vi "Teleop.vi"(10 "Match Info":T1={"Autonomous Elapsed Seconds"=0.0, "TeleOp Elapsed Seconds"=0.0, "Disabled Elapsed Seconds"=0.0, "Visited Autonomous"=FALSE, "Visited TeleOp"=FALSE, "Visited Disabled"=FALSE, "Autonomous Settings"={"Autonomous Style"=enum."Independent", "VI Refnum"=refnum}}, 11 "Call Context":T2) -> ()   [LabVIEW 2015]
doc: "This VI is called for each TeleOp packet received from the DS where the robot is not disabled. It is often used to read from the joysticks and update I/O or to update setpoints for timed control loops. It should complete and return within 20 milliseconds or it may miss DS packets."
uses:
  <vilib>/Rock Robotics/WPI/DriverStation/WPI_DriverStationDerivedRobotMode.ctl
  <vilib>/Rock Robotics/WPI/DriverStation/WPI_DriverStationMatch Info.ctl
  <vilib>/Rock Robotics/WPI/Solenoid/WPI_SolenoidValue.ctl
  <vilib>/Rock Robotics/Network Tables/NT Read Boolean.vi
  <vilib>/Rock Robotics/Network Tables/NT Read Number.vi
  <vilib>/Rock Robotics/WPI/Utilities/WPI_GetSetVariantRefNum.vi
  <vilib>/addons/control/pid/pid.llb/PID (DBL).vi
  <vilib>/Rock Robotics/WPI/Solenoid/WPI_SolenoidGetEnum.vi
  <vilib>/Rock Robotics/WPI/Solenoid/WPI_SolenoidSetEnum.vi
  <vilib>/addons/control/pid/NI_PID_pid.lvlib
panel:
  out "Sample Slider 0":dbl(slide) scale=0.0..5.0
  out "Sample Boolean 1":bool
  out "Sample Boolean 0":bool
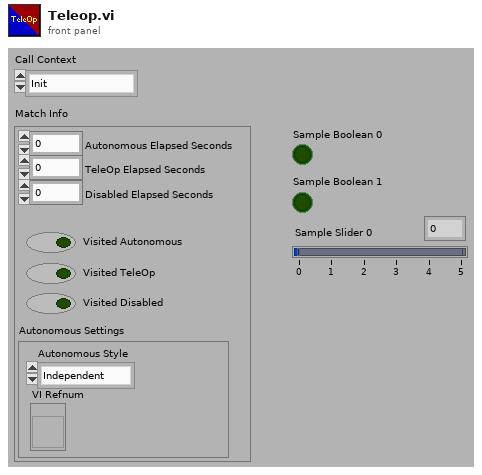
[diagram p1: front panel]
types:
  T1 = typedef "WPI_DriverStationMatch Info.ctl" = cluster{"Autonomous Elapsed Seconds":dbl, "TeleOp Elapsed Seconds":dbl, "Disabled Elapsed Seconds":dbl, "Visited Autonomous":bool, "Visited TeleOp":bool, "Visited Disabled":bool, "Autonomous Settings":cluster{"Autonomous Style":enum16{"Iterative", "Independent"}, "VI Refnum":refnum<vi>}}
  T2 = typedef "WPI_DriverStationDerivedRobotMode.ctl" = enum16{"Init", "Execute", "Stop"}
  T3 = typedef "WPI_SolenoidValue.ctl" = enum16{"Off", "On", "Forward", "Reverse"}
  T4 = typedef "WPI_JoystickDevRef.ctl" = cluster{"Device":T5}
  T5 = typedef "WPI_JoystickDeviceEnum.ctl" = enum16{"USB 0", "USB 1", "USB 2", "USB 3", "USB 4", "USB 5"}
  T6 = cluster{"Buttons[0]":bool, "Buttons[1]":bool, "Buttons[2]":bool, "Buttons[3]":bool, "Buttons[4]":bool, "Buttons[5]":bool, "Buttons[6]":bool, "Buttons[7]":bool, "Buttons[8]":bool}
  T7 = typedef "WPI_SolenoidDevRef.ctl" = cluster{"DevStatus":errorcluster, "Pneumatics Control Module":u8, "Forward Solenoid Channel":T8, "Reverse Solenoid Channel":T8}
  T8 = typedef "WPI_SolenoidChannel.ctl" = enum8{"Solenoid 0", "Solenoid 1", "Solenoid 2", "Solenoid 3", "Solenoid 4", "Solenoid 5", "Solenoid 6", "Solenoid 7", "Invalid"}
  T9 = cluster{"proportional gain (Kc)":dbl, "integral time (Ti, min)":dbl, "derivative time (Td, min)":dbl}
  T10 = cluster{"Axes[0]":dbl, "Axes[1]":dbl, "Axes[2]":dbl, "Axes[3]":dbl, "Axes[4]":dbl, "Axes[5]":dbl, "Axes[6]":dbl, "Axes[7]":dbl, "Axes[8]":dbl}
  T11 = typedef "WPI_RobotDriveDevRef.ctl" = cluster{"DevStatus":errorcluster, "Motors[]":T12[], "Square Inputs":bool, "Max Output":dbl}
  T12 = typedef "WPI_MotorControlDeviceRef.ctl" = cluster{"DeviceStatus":errorcluster, "Type":T13, "PWM":cluster{"PWM Channel":T14, "DeadBand":T15}, "CAN":cluster{"Device Number":u8, "Control Mode":T16, "Semaphore":T17, "Max Vout":dbl, "TalonSRX Control Mode":T18}, "Invert":bool}
  T13 = typedef "WPI_MotorControlType.ctl" = enum16{"PWM", "CAN", "CANTalonSRX"}
  T14 = typedef "FPGA_DIOPWMChannel.ctl" = enum8{"PWM 0", "PWM 1", "PWM 2", "PWM 3", "PWM 4", "PWM 5", "PWM 6", "PWM 7", "PWM 8", "PWM 9", "PWM MXP 0", "PWM MXP 1", "PWM MXP 2", "PWM MXP 3", "PWM MXP 4", "PWM MXP 5", "PWM MXP 6", "PWM MXP 7", "PWM MXP 8", "PWM MXP 9", "Invalid"}
  T15 = typedef "WPI_PWMDeadband.ctl" = cluster{"Name":string, "maxPositivePwm":i32, "minPositivePwm":i32, "centerPwm":i32, "maxNegativePwm":i32, "minNegativePwm":i32, "angularRange":u16}
  T16 = typedef "WPI_CANJaguar_ControlMode.ctl" = enum8{"Percent VBus", "Current", "Speed", "Position", "Voltage"}
  T17 = typedef "Semaphore RefNum" = refnum<k1>
  T18 = typedef "WPI_CANTalonSRX_APIControlMode.ctl" = enum8{"Percent VBus", "Speed", "Position", "Slave", "Unchanged / Invalid", "Voltage Compensation", "Current", "Motion Profile"}
  T19 = typedef "WPI_EncoderDevRef.ctl" = cluster{"DevStatus":errorcluster, "EncoderIndex":T20, "CounterIndex":T21, "DistancePerCount":dbl, "Decoding Type":T22}
  T20 = typedef "FPGA_EncoderIdx.ctl" = enum8{"Enc 0", "Enc 1", "Enc 2", "Enc 3", "Enc 4", "Enc 5", "Enc 6", "Enc 7", "Invalid"}
  T21 = typedef "FPGA_CounterCtrSystemIndex.ctl" = enum8{"Ctr 0", "Ctr 1", "Ctr 2", "Ctr 3", "Ctr 4", "Ctr 5", "Ctr 6", "Ctr 7", "Invalid"}
  T22 = typedef "WPI_EncoderType.ctl" = enum16{"1x", "2x", "4x"}
  T23 = typedef "WPI_CompressorDevRef.ctl" = cluster{"DevStatus":errorcluster, "Pneumatics Control Module":u8}
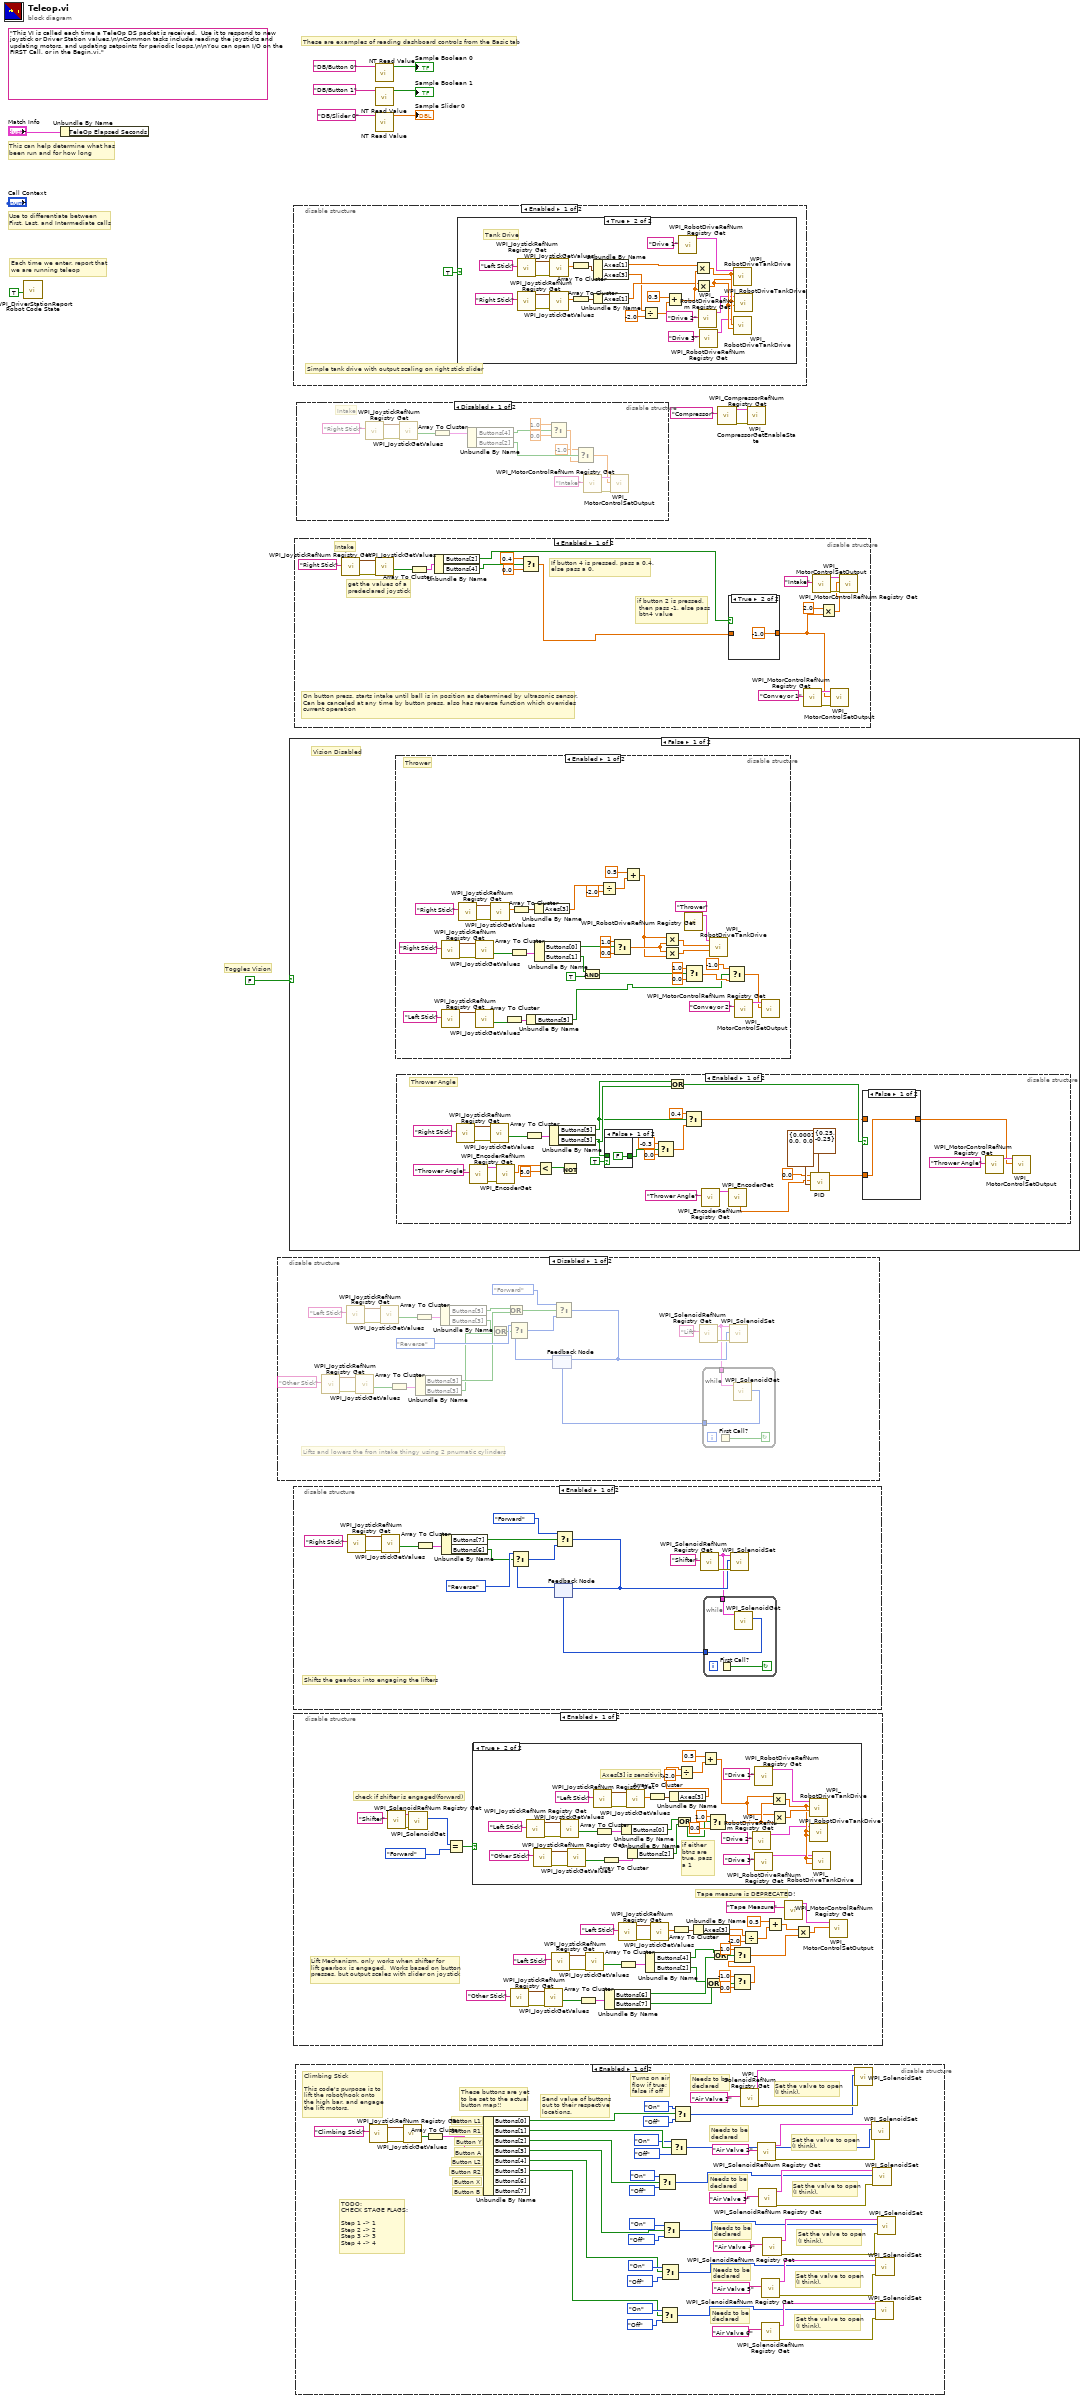
[diagram p0: block diagram]
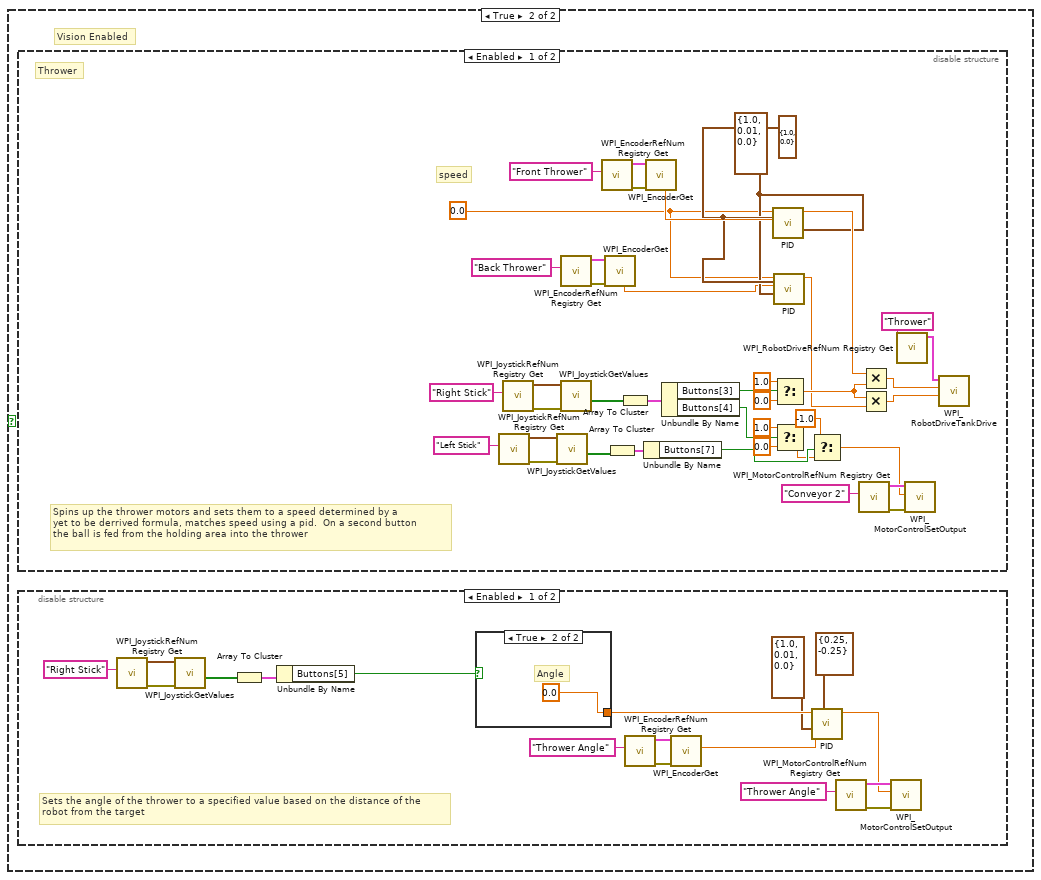
[diagram p11: hidden frame]
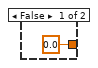
[diagram p12: hidden frame]
diagram:
  (unwired) "This VI is called each time a TeleOp DS packet is received.  Use it to respond to new joystick or Driver Station values.\n\nCommon tasks include reading the joysticks and updating motors, and updating setpoints for periodic loops.\n\nYou can open I/O on the FIRST Call, or in the Begin.vi."
  # "Toggles Vision"
  # "These are examples of reading dashboard controls from the Basic tab"
  # "Each time we enter, report that\nwe are running teleop"
  # "Use to differentiate between\nFirst, Last, and Intermediate calls"
  # "This can help determine what has\nbeen run and for how long"
  n1 = call <vilib>:"WPI_DriverStationReport Robot Code State.vi"("TeleOp"=TRUE ("Autonomous")) -> ()  [unwired: 10 in, 1 out]
  n2 = Unbundle By Name("Match Info") -> ()  [unwired: 1 out]
  n3 = disable-structure shown="Disabled" {
    frame Disabled {
      # "Lifts and lowers the fron intake thingy using 2 pnumatic cylinders"
      n4 = call <vilib>:"WPI_JoystickRefNum Registry Get.vi"("refnum name"="Other Stick") -> ("error out"=w23:errorcluster, "JoystickDevRef"=w22:T4)  [unwired: 9 in]
      n5 = call <vilib>:"WPI_JoystickRefNum Registry Get.vi"("refnum name"="Left Stick") -> ("error out"=w37:errorcluster, "JoystickDevRef"=w36:T4)  [unwired: 9 in]
      n6 = call <vilib>:"WPI_JoystickGetValues.vi"("error in (no error)"=w23, "JoystickDevRef"=w22) -> ("Buttons"=w20:bool[])  [unwired: 5 in, 4 out]
      n7 = call <vilib>:"WPI_JoystickGetValues.vi"("error in (no error)"=w37, "JoystickDevRef"=w36) -> ("Buttons"=w34:bool[])  [unwired: 5 in, 4 out]
      n8 = Array To Cluster(array=w20) -> (cluster=w19:T6)
      n9 = Array To Cluster(array=w34) -> (cluster=w33:T6)
      n10 = Unbundle By Name(w19) -> ("Buttons[5]"=w16:bool, "Buttons[3]"=w14:bool)
      n11 = Unbundle By Name(w33) -> ("Buttons[5]"=w18:bool, "Buttons[3]"=w13:bool)
      n12 = Or(x=w13, y=w14) -> (x .or. y?=w15:bool)
      n13 = Or(x=w18, y=w16) -> (x .or. y?=w17:bool)
      n14 = call <vilib>:"WPI_SolenoidRefNum Registry Get.vi"("refnum name"="Lift") -> ("error out"=w31:errorcluster, "SolenoidDevRef"=w25:T7)  [unwired: 9 in]
      n15 = while {
        tunnel: w25 -> [w39]
        tunnel: [w38] -> w24
        stop <- w40 continue-if-true
        n16 = First Call?() -> (First Call?: T/F=w40:bool)
        n17 = call-poly <vilib>:"WPI_SolenoidGet.vi"("SolenoidDevRef"=w39) -> ("Value"=w38:T3)  [unwired: 8 in, 2 out]
      }
      n18 = feedback #1(w24) -> (w26:T3)
      n19 = Select(t=WPI_SolenoidValue."Reverse" ("Value"), s=w15, f=w26) -> (s? t:f=w28:T3)
      n20 = Select(t=WPI_SolenoidValue."Forward" ("Value"), s=w17, f=w28) -> (s? t:f=w27:T3)
      n21 = feedback-in #1(w27) -> ()
      n22 = call-poly <vilib>:"WPI_SolenoidSet.vi"("error in (no error)"=w31, "Value"=w27, "SolenoidDevRef"=w25) -> ()  [unwired: 7 in, 2 out]
    }
    frame Enabled {
    }
  }
  n23 = case shown="False" FALSE {
    frame False {
      # "Vision Disabled"
      n24 = disable-structure shown="Enabled" {
        frame Enabled {
          # "Thrower"
          n25 = call <vilib>:"WPI_JoystickRefNum Registry Get.vi"("refnum name"="Right Stick") -> ("error out"=w113:errorcluster, "JoystickDevRef"=w112:T4)  [unwired: 9 in]
          n26 = call <vilib>:"WPI_JoystickRefNum Registry Get.vi"("refnum name"="Left Stick") -> ("JoystickDevRef"=w84:T4)  [unwired: 9 in, 1 out]
          n27 = call <vilib>:"WPI_JoystickRefNum Registry Get.vi"("refnum name"="Right Stick") -> ("error out"=w96:errorcluster, "JoystickDevRef"=w95:T4)  [unwired: 9 in]
          n28 = call <vilib>:"WPI_JoystickGetValues.vi"("error in (no error)"=w113, "JoystickDevRef"=w112) -> ("Buttons"=w110:bool[])  [unwired: 5 in, 4 out]
          n29 = call <vilib>:"WPI_JoystickGetValues.vi"("JoystickDevRef"=w84) -> ("Buttons"=w82:bool[])  [unwired: 6 in, 4 out]
          n30 = call <vilib>:"WPI_JoystickGetValues.vi"("error in (no error)"=w96, "JoystickDevRef"=w95) -> ("Axes"=w94:dbl[])  [unwired: 5 in, 4 out]
          n31 = Array To Cluster(array=w82) -> (cluster=w81:T6)
          n32 = Array To Cluster(array=w110) -> (cluster=w109:T6)
          n33 = Array To Cluster(array=w94) -> (cluster=w93:T10)
          n34 = Unbundle By Name(w81) -> ("Buttons[5]"=w76:bool)
          n35 = Unbundle By Name(w93) -> ("Axes[3]"=w89:dbl)
          n36 = Unbundle By Name(w109) -> ("Buttons[0]"=w108:bool, "Buttons[1]"=w86:bool)
          n37 = And(x=w86, y=TRUE) -> (x .and. y?=w80:bool)
          n38 = Divide(x=w89, y=-2.0) -> (x/y=w91:dbl)
          n39 = Select(t=1.0, s=w108, f=0.0) -> (s? t:f=w105:dbl)
          n40 = Add(x=0.5, y=w91) -> (x+y=w87:dbl)
          n41 = Multiply(x=w87, y=w105) -> (x*y=w103:dbl)
          n42 = Multiply(x=w105, y=w87) -> (x*y=w104:dbl)
          n43 = call <vilib>:"WPI_RobotDriveRefNum Registry Get.vi"("refnum name"="Thrower") -> ("RobotDriveDevRef"=w102:T11)  [unwired: 9 in, 1 out]
          n44 = Select(t=1.0, s=w80, f=0.0) -> (s? t:f=w79:dbl)
          n45 = call <vilib>:"WPI_RobotDriveTankDrive.vi"("Right axis value"=w104, "Left axis value"=w103, "RobotDriveDevRef"=w102) -> ()  [unwired: 6 in, 3 out]
          n46 = Select(t=-1.0, s=w76, f=w79) -> (s? t:f=w77:dbl)
          n47 = call <vilib>:"WPI_MotorControlRefNum Registry Get.vi"("refnum name"="Conveyor 2") -> ("MotorControlDevRef"=w100:T12)  [unwired: 9 in, 1 out]
          n48 = call <vilib>:"WPI_MotorControlSetOutput.vi"("Output"=w77, "MotorControlDevRef"=w100) -> ()  [unwired: 7 in, 3 out]
        }
        frame Disabled {
        }
      }
      n49 = disable-structure shown="Enabled" {
        frame Enabled {
          # "Thrower Angle"
          n50 = call <vilib>:"WPI_JoystickRefNum Registry Get.vi"("refnum name"="Right Stick") -> ("error out"=w71:errorcluster, "JoystickDevRef"=w70:T4)  [unwired: 9 in]
          n51 = call <vilib>:"WPI_EncoderRefNum Registry Get.vi"("refnum name"="Thrower Angle") -> ("error out"=w63:errorcluster, "EncoderDevRef"=w61:T19)  [unwired: 9 in]
          n52 = call <vilib>:"WPI_JoystickGetValues.vi"("error in (no error)"=w71, "JoystickDevRef"=w70) -> ("Buttons"=w68:bool[])  [unwired: 5 in, 4 out]
          n53 = call <vilib>:"WPI_EncoderGet.vi"("error in (no error)"=w63, "EncoderDevRef"=w61) -> ("Distance"=w60:dbl)  [unwired: 4 in, 5 out]
          n54 = Array To Cluster(array=w68) -> (cluster=w67:T6)
          n55 = Less?(x=w60, y=5.0) -> (x < y?=w58:bool)
          n56 = Unbundle By Name(w67) -> ("Buttons[5]"=w47:bool, "Buttons[3]"=w48:bool)
          n57 = Not(x=w58) -> ()  [unwired: 1 out]
          n58 = case shown="False" TRUE {
            tunnel: w48 -> [_ w75]
            tunnel: [FALSE ("Buttons[6]") w75] -> w57
            frame False {
            }
            frame True {
            }
          }
          n59 = Select(t=-0.3, s=w57, f=0.0) -> (s? t:f=w56:dbl)
          n60 = Or(x=w47, y=w48) -> (x .or. y?=w46:bool)
          n61 = Select(t=0.4, s=w47, f=w56) -> (s? t:f=w45:dbl)
          n62 = call <vilib>:"WPI_EncoderRefNum Registry Get.vi"("refnum name"="Thrower Angle") -> ("EncoderDevRef"=w52:T19)  [unwired: 9 in, 1 out]
          n63 = call <vilib>:"WPI_EncoderGet.vi"("EncoderDevRef"=w52) -> ("Rate"=w41:dbl)  [unwired: 5 in, 5 out]
          n64 = call-poly <vilib>:"PID.vi"("output range"=cluster{"output high":dbl, "output low":dbl} {"output high"=0.25, "output low"=-0.25}, "PID gains"=T9 {"proportional gain (Kc)"=0.0001, "integral time (Ti, min)"=0.0, "derivative time (Td, min)"=0.0}, "process variable"=w41, "setpoint"=0.0) -> ("output"=w43:dbl)  [unwired: 6 in, 1 out]
          n65 = case shown="False" w46 {
            tunnel: [w72 w73] -> w44
            tunnel: w45 -> [_ w73]
            tunnel: w43 -> [w72 _]
            frame False {
            }
            frame True {
            }
          }
          n66 = call <vilib>:"WPI_MotorControlRefNum Registry Get.vi"("refnum name"="Thrower Angle") -> ("MotorControlDevRef"=w54:T12)  [unwired: 9 in, 1 out]
          n67 = call <vilib>:"WPI_MotorControlSetOutput.vi"("Output"=w44, "MotorControlDevRef"=w54) -> ()  [unwired: 7 in, 3 out]
        }
        frame Disabled {
        }
      }
    }
    frame True {
      # "Vision Enabled"
      n68 = disable-structure shown="Enabled" {
        frame Enabled {
          w153 = 0.0 ("setpoint")
          w154 = T9 {"proportional gain (Kc)"=1.0, "integral time (Ti, min)"=0.01, "derivative time (Td, min)"=0.0} ("PID gains")
          w155 = cluster{"output high":dbl, "output low":dbl} {"output high"=1.0, "output low"=0.0} ("output range")
          # "Spins up the thrower motors and sets them to a speed determined by a \nyet to be derrived formula, matches speed using a pid.  On a second button\nthe ball is fed from the holding area into the thrower"
          # "Thrower"
          # "speed"
          n69 = call <vilib>:"WPI_JoystickRefNum Registry Get.vi"("refnum name"="Left Stick") -> ("error out"=w141:errorcluster, "JoystickDevRef"=w140:T4)  [unwired: 9 in]
          n70 = call <vilib>:"WPI_JoystickRefNum Registry Get.vi"("refnum name"="Right Stick") -> ("error out"=w173:errorcluster, "JoystickDevRef"=w172:T4)  [unwired: 9 in]
          n71 = call <vilib>:"WPI_JoystickGetValues.vi"("error in (no error)"=w141, "JoystickDevRef"=w140) -> ("Buttons"=w138:bool[])  [unwired: 5 in, 4 out]
          n72 = call <vilib>:"WPI_EncoderRefNum Registry Get.vi"("refnum name"="Back Thrower") -> ("error out"=w152:errorcluster, "EncoderDevRef"=w151:T19)  [unwired: 9 in]
          n73 = call <vilib>:"WPI_JoystickGetValues.vi"("error in (no error)"=w173, "JoystickDevRef"=w172) -> ("Buttons"=w170:bool[])  [unwired: 5 in, 4 out]
          n74 = call <vilib>:"WPI_EncoderRefNum Registry Get.vi"("refnum name"="Front Thrower") -> ("error out"=w160:errorcluster, "EncoderDevRef"=w159:T19)  [unwired: 9 in]
          n75 = call <vilib>:"WPI_EncoderGet.vi"("error in (no error)"=w152, "EncoderDevRef"=w151) -> ("Rate"=w149:dbl)  [unwired: 4 in, 5 out]
          n76 = Array To Cluster(array=w138) -> (cluster=w137:T6)
          n77 = Array To Cluster(array=w170) -> (cluster=w169:T6)
          n78 = Unbundle By Name(w137) -> ("Buttons[7]"=w136:bool)
          n79 = call <vilib>:"WPI_EncoderGet.vi"("error in (no error)"=w160, "EncoderDevRef"=w159) -> ("Rate"=w157:dbl)  [unwired: 4 in, 5 out]
          n80 = Unbundle By Name(w169) -> ("Buttons[3]"=w168:bool, "Buttons[4]"=w143:bool)
          n81 = call-poly <vilib>:"PID.vi"("output range"=w155, "PID gains"=w154, "process variable"=w157, "setpoint"=w153) -> ("output"=w156:dbl)  [unwired: 6 in, 1 out]
          n82 = call-poly <vilib>:"PID.vi"("output range"=w155, "PID gains"=w154, "process variable"=w149, "setpoint"=w153) -> ("output"=w148:dbl)  [unwired: 6 in, 1 out]
          n83 = Select(t=1.0, s=w168, f=0.0) -> (s? t:f=w165:dbl)
          n84 = Select(t=1.0, s=w143, f=0.0) -> (s? t:f=w135:dbl)
          n85 = Select(t=-1.0, s=w136, f=w135) -> (s? t:f=w133:dbl)
          n86 = call <vilib>:"WPI_MotorControlRefNum Registry Get.vi"("refnum name"="Conveyor 2") -> ("error out"=w147:errorcluster, "MotorControlDevRef"=w145:T12)  [unwired: 9 in]
          n87 = Multiply(x=w156, y=w165) -> (x*y=w163:dbl)
          n88 = Multiply(x=w165, y=w148) -> (x*y=w164:dbl)
          n89 = call <vilib>:"WPI_RobotDriveRefNum Registry Get.vi"("refnum name"="Thrower") -> ("RobotDriveDevRef"=w162:T11)  [unwired: 9 in, 1 out]
          n90 = call <vilib>:"WPI_MotorControlSetOutput.vi"("error in (no error)"=w147, "Output"=w133, "MotorControlDevRef"=w145) -> ()  [unwired: 6 in, 3 out]
          n91 = call <vilib>:"WPI_RobotDriveTankDrive.vi"("Right axis value"=w164, "Left axis value"=w163, "RobotDriveDevRef"=w162) -> ()  [unwired: 6 in, 3 out]
        }
        frame Disabled {
        }
      }
      n92 = disable-structure shown="Enabled" {
        frame Enabled {
          # "Sets the angle of the thrower to a specified value based on the distance of the\nrobot from the target"
          n93 = call <vilib>:"WPI_JoystickRefNum Registry Get.vi"("refnum name"="Right Stick") -> ("error out"=w120:errorcluster, "JoystickDevRef"=w119:T4)  [unwired: 9 in]
          n94 = call <vilib>:"WPI_JoystickGetValues.vi"("error in (no error)"=w120, "JoystickDevRef"=w119) -> ("Buttons"=w117:bool[])  [unwired: 5 in, 4 out]
          n95 = Array To Cluster(array=w117) -> (cluster=w116:T6)
          n96 = Unbundle By Name(w116) -> ("Buttons[5]"=w115:bool)
          n97 = case shown="True" w115 {
            tunnel: [0.0 ("setpoint") 0.0 ("setpoint")] -> w128
            frame False {
            }
            frame True {
              # "Angle"
            }
          }
          n98 = call <vilib>:"WPI_EncoderRefNum Registry Get.vi"("refnum name"="Thrower Angle") -> ("error out"=w130:errorcluster, "EncoderDevRef"=w129:T19)  [unwired: 9 in]
          n99 = call <vilib>:"WPI_EncoderGet.vi"("error in (no error)"=w130, "EncoderDevRef"=w129) -> ("Distance"=w127:dbl)  [unwired: 4 in, 5 out]
          n100 = call-poly <vilib>:"PID.vi"("output range"=cluster{"output high":dbl, "output low":dbl} {"output high"=0.25, "output low"=-0.25}, "PID gains"=T9 {"proportional gain (Kc)"=1.0, "integral time (Ti, min)"=0.01, "derivative time (Td, min)"=0.0}, "process variable"=w127, "setpoint"=w128) -> ("output"=w121:dbl)  [unwired: 6 in, 1 out]
          n101 = call <vilib>:"WPI_MotorControlRefNum Registry Get.vi"("refnum name"="Thrower Angle") -> ("error out"=w123:errorcluster, "MotorControlDevRef"=w122:T12)  [unwired: 9 in]
          n102 = call <vilib>:"WPI_MotorControlSetOutput.vi"("error in (no error)"=w123, "Output"=w121, "MotorControlDevRef"=w122) -> ()  [unwired: 6 in, 3 out]
        }
        frame Disabled {
        }
      }
    }
  }
  n103 = disable-structure shown="Enabled" {
    frame Enabled {
      # "Shifts the gearbox into engaging the lifters"
      n104 = call <vilib>:"WPI_JoystickRefNum Registry Get.vi"("refnum name"="Right Stick") -> ("error out"=w189:errorcluster, "JoystickDevRef"=w188:T4)  [unwired: 9 in]
      n105 = call <vilib>:"WPI_JoystickGetValues.vi"("error in (no error)"=w189, "JoystickDevRef"=w188) -> ("Buttons"=w186:bool[])  [unwired: 5 in, 4 out]
      n106 = Array To Cluster(array=w186) -> (cluster=w185:T6)
      n107 = Unbundle By Name(w185) -> ("Buttons[7]"=w179:bool, "Buttons[6]"=w180:bool)
      n108 = call <vilib>:"WPI_SolenoidRefNum Registry Get.vi"("refnum name"="Shifter") -> ("error out"=w183:errorcluster, "SolenoidDevRef"=w175:T7)  [unwired: 9 in]
      n109 = while {
        tunnel: w175 -> [w191]
        tunnel: [w190] -> w174
        stop <- w192 continue-if-true
        n110 = First Call?() -> (First Call?: T/F=w192:bool)
        n111 = call-poly <vilib>:"WPI_SolenoidGet.vi"("SolenoidDevRef"=w191) -> ("Value"=w190:T3)  [unwired: 8 in, 2 out]
      }
      n112 = feedback #2(w174) -> (w176:T3)
      n113 = Select(t=WPI_SolenoidValue."Reverse" ("Value"), s=w180, f=w176) -> (s? t:f=w178:T3)
      n114 = Select(t=WPI_SolenoidValue."Forward" ("Value"), s=w179, f=w178) -> (s? t:f=w177:T3)
      n115 = feedback-in #2(w177) -> ()
      n116 = call-poly <vilib>:"WPI_SolenoidSet.vi"("error in (no error)"=w183, "Value"=w177, "SolenoidDevRef"=w175) -> ()  [unwired: 7 in, 2 out]
    }
    frame Disabled {
    }
  }
  n117 = disable-structure shown="Enabled" {
    frame Enabled {
      # "Simple tank drive with output scaling on right stick slider"
      n118 = case shown="True" TRUE {
        frame False {
        }
        frame True {
          # "Tank Drive"
          n119 = call <vilib>:"WPI_JoystickRefNum Registry Get.vi"("refnum name"="Left Stick") -> ("error out"=w217:errorcluster, "JoystickDevRef"=w216:T4)  [unwired: 9 in]
          n120 = call <vilib>:"WPI_JoystickRefNum Registry Get.vi"("refnum name"="Right Stick") -> ("error out"=w212:errorcluster, "JoystickDevRef"=w211:T4)  [unwired: 9 in]
          n121 = call <vilib>:"WPI_JoystickGetValues.vi"("error in (no error)"=w217, "JoystickDevRef"=w216) -> ("Axes"=w215:dbl[])  [unwired: 5 in, 4 out]
          n122 = call <vilib>:"WPI_JoystickGetValues.vi"("error in (no error)"=w212, "JoystickDevRef"=w211) -> ("Axes"=w210:dbl[])  [unwired: 5 in, 4 out]
          n123 = Array To Cluster(array=w215) -> (cluster=w214:T10)
          n124 = Array To Cluster(array=w210) -> (cluster=w209:T10)
          n125 = Unbundle By Name(w214) -> ("Axes[1]"=w203:dbl, "Axes[3]"=w194:dbl)
          n126 = Unbundle By Name(w209) -> ("Axes[1]"=w204:dbl)
          n127 = Divide(x=w194, y=-2.0) -> (x/y=w207:dbl)
          n128 = Add(x=0.5, y=w207) -> (x+y=w205:dbl)
          n129 = call <vilib>:"WPI_RobotDriveRefNum Registry Get.vi"("refnum name"="Drive 1") -> ("RobotDriveDevRef"=w202:T11)  [unwired: 9 in, 1 out]
          n130 = Multiply(x=w203, y=w205) -> (x*y=w200:dbl)
          n131 = Multiply(x=w204, y=w205) -> (x*y=w199:dbl)
          n132 = call <vilib>:"WPI_RobotDriveRefNum Registry Get.vi"("refnum name"="Drive 2") -> ("RobotDriveDevRef"=w197:T11)  [unwired: 9 in, 1 out]
          n133 = call <vilib>:"WPI_RobotDriveRefNum Registry Get.vi"("refnum name"="Drive 3") -> ("RobotDriveDevRef"=w195:T11)  [unwired: 9 in, 1 out]
          n134 = call <vilib>:"WPI_RobotDriveTankDrive.vi"("Right axis value"=w199, "Left axis value"=w200, "RobotDriveDevRef"=w202) -> ()  [unwired: 6 in, 3 out]
          n135 = call <vilib>:"WPI_RobotDriveTankDrive.vi"("Right axis value"=w199, "Left axis value"=w200, "RobotDriveDevRef"=w195) -> ()  [unwired: 6 in, 3 out]
          n136 = call <vilib>:"WPI_RobotDriveTankDrive.vi"("Right axis value"=w199, "Left axis value"=w200, "RobotDriveDevRef"=w197) -> ()  [unwired: 6 in, 3 out]
        }
      }
    }
    frame Disabled {
    }
  }
  n137 = disable-structure shown="Enabled" {
    frame Enabled {
      # "Tape measure is DEPRECATED!"
      # "check if shifter is engaged(forward)"
      # "Lift Mechanism, only works when shifter for\nlift gearbox is engaged.  Works based on button\npresses, but output scales with slider on joystick"
      n138 = call <vilib>:"WPI_SolenoidRefNum Registry Get.vi"("refnum name"="Shifter") -> ("error out"=w257:errorcluster, "SolenoidDevRef"=w256:T7)  [unwired: 9 in]
      n139 = call-poly <vilib>:"WPI_SolenoidGet.vi"("error in (no error)"=w257, "SolenoidDevRef"=w256) -> ("Value"=w254:T3)  [unwired: 7 in, 2 out]
      n140 = Equal?(x=w254, y=WPI_SolenoidValue."Forward") -> (x = y?=w255:bool)
      n141 = case shown="True" w255 {
        frame False {
        }
        frame True {
          # "Axes[3] is sensitivity"
          # "if either btns are true, pass a 1"
          n142 = call <vilib>:"WPI_JoystickRefNum Registry Get.vi"("refnum name"="Left Stick") -> ("error out"=w288:errorcluster, "JoystickDevRef"=w289:T4)  [unwired: 9 in]
          n143 = call <vilib>:"WPI_JoystickRefNum Registry Get.vi"("refnum name"="Other Stick") -> ("error out"=w271:errorcluster, "JoystickDevRef"=w270:T4)  [unwired: 9 in]
          n144 = call <vilib>:"WPI_JoystickGetValues.vi"("error in (no error)"=w288, "JoystickDevRef"=w289) -> ("Buttons"=w291:bool[])  [unwired: 5 in, 4 out]
          n145 = call <vilib>:"WPI_JoystickGetValues.vi"("error in (no error)"=w271, "JoystickDevRef"=w270) -> ("Buttons"=w268:bool[])  [unwired: 5 in, 4 out]
          n146 = call <vilib>:"WPI_JoystickRefNum Registry Get.vi"("refnum name"="Left Stick") -> ("error out"=w286:errorcluster, "JoystickDevRef"=w285:T4)  [unwired: 9 in]
          n147 = Array To Cluster(array=w291) -> (cluster=w292:T6)
          n148 = Array To Cluster(array=w268) -> (cluster=w267:T6)
          n149 = Unbundle By Name(w292) -> ("Buttons[0]"=w265:bool)
          n150 = call <vilib>:"WPI_JoystickGetValues.vi"("error in (no error)"=w286, "JoystickDevRef"=w285) -> ("Axes"=w284:dbl[])  [unwired: 5 in, 4 out]
          n151 = Unbundle By Name(w267) -> ("Buttons[2]"=w264:bool)
          n152 = Array To Cluster(array=w284) -> (cluster=w283:T10)
          n153 = Unbundle By Name(w283) -> ("Axes[3]"=w274:dbl)
          n154 = Or(x=w265, y=w264) -> (x .or. y?=w266:bool)
          n155 = Divide(x=w274, y=-2.0) -> (x/y=w277:dbl)
          n156 = Add(x=0.5, y=w277) -> (x+y=w273:dbl)
          n157 = Select(t=1.0, s=w266, f=0.0) -> (s? t:f=w278:dbl)
          n158 = call <vilib>:"WPI_RobotDriveRefNum Registry Get.vi"("refnum name"="Drive 2") -> ("RobotDriveDevRef"=w259:T11)  [unwired: 9 in, 1 out]
          n159 = call <vilib>:"WPI_RobotDriveRefNum Registry Get.vi"("refnum name"="Drive 1") -> ("RobotDriveDevRef"=w282:T11)  [unwired: 9 in, 1 out]
          n160 = call <vilib>:"WPI_RobotDriveRefNum Registry Get.vi"("refnum name"="Drive 3") -> ("RobotDriveDevRef"=w260:T11)  [unwired: 9 in, 1 out]
          n161 = Multiply(x=w273, y=w278) -> (x*y=w261:dbl)
          n162 = Multiply(x=w273, y=w278) -> (x*y=w280:dbl)
          n163 = call <vilib>:"WPI_RobotDriveTankDrive.vi"("Right axis value"=w280, "Left axis value"=w261, "RobotDriveDevRef"=w282) -> ()  [unwired: 6 in, 3 out]
          n164 = call <vilib>:"WPI_RobotDriveTankDrive.vi"("Right axis value"=w261, "Left axis value"=w261, "RobotDriveDevRef"=w259) -> ()  [unwired: 6 in, 3 out]
          n165 = call <vilib>:"WPI_RobotDriveTankDrive.vi"("Right axis value"=w261, "Left axis value"=w261, "RobotDriveDevRef"=w260) -> ()  [unwired: 6 in, 3 out]
        }
      }
      n166 = call <vilib>:"WPI_JoystickRefNum Registry Get.vi"("refnum name"="Other Stick") -> ("error out"=w229:errorcluster, "JoystickDevRef"=w220:T4)  [unwired: 9 in]
      n167 = call <vilib>:"WPI_JoystickGetValues.vi"("error in (no error)"=w229, "JoystickDevRef"=w220) -> ("Buttons"=w227:bool[])  [unwired: 5 in, 4 out]
      n168 = call <vilib>:"WPI_JoystickRefNum Registry Get.vi"("refnum name"="Left Stick") -> ("error out"=w248:errorcluster, "JoystickDevRef"=w249:T4)  [unwired: 9 in]
      n169 = Array To Cluster(array=w227) -> (cluster=w226:T6)
      n170 = call <vilib>:"WPI_JoystickGetValues.vi"("error in (no error)"=w248, "JoystickDevRef"=w249) -> ("Buttons"=w251:bool[])  [unwired: 5 in, 4 out]
      n171 = Unbundle By Name(w226) -> ("Buttons[6]"=w224:bool, "Buttons[7]"=w221:bool)
      n172 = call <vilib>:"WPI_JoystickRefNum Registry Get.vi"("refnum name"="Left Stick") -> ("error out"=w246:errorcluster, "JoystickDevRef"=w245:T4)  [unwired: 9 in]
      n173 = Array To Cluster(array=w251) -> (cluster=w252:T6)
      n174 = Unbundle By Name(w252) -> ("Buttons[4]"=w225:bool, "Buttons[2]"=w222:bool)
      n175 = call <vilib>:"WPI_JoystickGetValues.vi"("error in (no error)"=w246, "JoystickDevRef"=w245) -> ("Axes"=w244:dbl[])  [unwired: 5 in, 4 out]
      n176 = Array To Cluster(array=w244) -> (cluster=w243:T10)
      n177 = Unbundle By Name(w243) -> ("Axes[3]"=w232:dbl)
      n178 = Or(x=w222, y=w221) -> (x .or. y?=w223:bool)
      n179 = Or(x=w225, y=w224) -> (x .or. y?=w219:bool)
      n180 = Select(t=-1.0, s=w223, f=0.0) -> (s? t:f=w240:dbl)
      n181 = Select(t=1.0, s=w219, f=w240) -> (s? t:f=w239:dbl)
      n182 = Divide(x=w232, y=-2.0) -> (x/y=w235:dbl)
      n183 = Add(x=0.5, y=w235) -> (x+y=w231:dbl)
      n184 = call <vilib>:"WPI_MotorControlRefNum Registry Get.vi"("refnum name"="Tape Measure") -> ("MotorControlDevRef"=w237:T12)  [unwired: 9 in, 1 out]
      n185 = Multiply(x=w231, y=w239) -> (x*y=w236:dbl)
      n186 = call <vilib>:"WPI_MotorControlSetOutput.vi"("Output"=w236, "MotorControlDevRef"=w237) -> ()  [unwired: 7 in, 3 out]
    }
    frame Disabled {
    }
  }
  n187 = disable-structure shown="Enabled" {
    frame Enabled {
      # "if button 2 is pressed,\n then pass -1, else pass\n btn4 value"
      # "get the values of a\npredeclared joystick"
      # "If button 4 is pressed, pass a 0.4.\nelse pass a 0."
      # "On button press, starts intake until ball is in position as determined by ultrasonic sensor.\nCan be canceled at any time by button press, also has reverse function which overrides \ncurrent operation"
      # "Intake"
      n188 = call <vilib>:"WPI_JoystickRefNum Registry Get.vi"("refnum name"="Right Stick") -> ("error out"=w311:errorcluster, "JoystickDevRef"=w310:T4)  [unwired: 9 in]
      n189 = call <vilib>:"WPI_JoystickGetValues.vi"("error in (no error)"=w311, "JoystickDevRef"=w310) -> ("Buttons"=w308:bool[])  [unwired: 5 in, 4 out]
      n190 = Array To Cluster(array=w308) -> (cluster=w307:T6)
      n191 = Unbundle By Name(w307) -> ("Buttons[2]"=w302:bool, "Buttons[4]"=w306:bool)
      n192 = Select(t=0.4, s=w306, f=0.0) -> (s? t:f=w293:dbl)
      n193 = case shown="True" w302 {
        tunnel: [w312 -1.0 ("t")] -> w296
        tunnel: w293 -> [w312 _]
        frame False {
        }
        frame True {
        }
      }
      n194 = call <vilib>:"WPI_MotorControlRefNum Registry Get.vi"("refnum name"="Conveyor 1") -> ("error out"=w305:errorcluster, "MotorControlDevRef"=w303:T12)  [unwired: 9 in]
      n195 = call <vilib>:"WPI_MotorControlRefNum Registry Get.vi"("refnum name"="Intake") -> ("error out"=w298:errorcluster, "MotorControlDevRef"=w297:T12)  [unwired: 9 in]
      n196 = Multiply(x=2.0, y=w296) -> (x*y=w294:dbl)
      n197 = call <vilib>:"WPI_MotorControlSetOutput.vi"("error in (no error)"=w305, "Output"=w296, "MotorControlDevRef"=w303) -> ()  [unwired: 6 in, 3 out]
      n198 = call <vilib>:"WPI_MotorControlSetOutput.vi"("error in (no error)"=w298, "Output"=w294, "MotorControlDevRef"=w297) -> ()  [unwired: 6 in, 3 out]
    }
    frame Disabled {
    }
  }
  n199 = disable-structure shown="Enabled" {
    frame Enabled {
      # "Button B"
      # "Set the valve to open\n(I think)."
      # "Needs to be\ndeclared"
      # "Set the valve to open\n(I think)."
      # "Needs to be\ndeclared"
      # "Button X"
      # "Button R2"
      # "Button L2"
      # "Set the valve to open\n(I think)."
      # "Needs to be\ndeclared"
      # "Set the valve to open\n(I think)."
      # "Needs to be\ndeclared"
      # "Set the valve to open\n(I think)."
      # "Needs to be\ndeclared"
      # "Set the valve to open\n(I think)."
      # "Send value of buttons\nout to their respective\nlocations."
      # "Turns on air\nflow if true; \nfalse if off"
      # "Needs to be\ndeclared"
      # "Climbing Stick\n\nThis code's purpose is to\nlift the robot/hook onto \nthe high bar, and engage\nthe lift motors."
      # "These buttons are yet\nto be set to the actual\nbutton map!!"
      # "TODO: \nCHECK STAGE FLAGS:\n\nStep 1 -> 1\nStep 2 -> 2\nStep 3 -> 3\nStep 4 -> 4"
      # "Button A"
      # "Button Y"
      # "Button R1"
      # "Button L1"
      n200 = call <vilib>:"WPI_JoystickRefNum Registry Get.vi"("refnum name"="Climbing Stick") -> ("error out"=w360:errorcluster, "JoystickDevRef"=w358:T4)  [unwired: 9 in]
      n201 = call <vilib>:"WPI_JoystickGetValues.vi"("error in (no error)"=w360, "JoystickDevRef"=w358) -> ("Buttons"=w356:bool[])  [unwired: 5 in, 4 out]
      n202 = Array To Cluster(array=w356) -> (cluster=w357:T6)
      n203 = Unbundle By Name(w357) -> ("Buttons[0]"=w351:bool, "Buttons[1]"=w343:bool, "Buttons[2]"=w336:bool, "Buttons[3]"=w329:bool, "Buttons[4]"=w321:bool, "Buttons[5]"=w314:bool)  [unwired: 2 out]
      n204 = Select(t=WPI_SolenoidValue."On" ("Value"), s=w336, f=WPI_SolenoidValue."Off" ("Value")) -> (s? t:f=w337:T3)
      n205 = Select(t=WPI_SolenoidValue."On" ("Value"), s=w314, f=WPI_SolenoidValue."Off" ("Value")) -> (s? t:f=w317:T3)
      n206 = Select(t=WPI_SolenoidValue."On" ("Value"), s=w321, f=WPI_SolenoidValue."Off" ("Value")) -> (s? t:f=w324:T3)
      n207 = Select(t=WPI_SolenoidValue."On" ("Value"), s=w329, f=WPI_SolenoidValue."Off" ("Value")) -> (s? t:f=w332:T3)
      n208 = Select(t=WPI_SolenoidValue."On" ("Value"), s=w343, f=WPI_SolenoidValue."Off" ("Value")) -> (s? t:f=w344:T3)
      n209 = Select(t=WPI_SolenoidValue."On" ("Value"), s=w351, f=WPI_SolenoidValue."Off" ("Value")) -> (s? t:f=w350:T3)
      n210 = call <vilib>:"WPI_SolenoidRefNum Registry Get.vi"("refnum name"="Air Valve 1") -> ("error out"=w355:errorcluster, "SolenoidDevRef"=w354:T7)  [unwired: 9 in]
      n211 = call <vilib>:"WPI_SolenoidRefNum Registry Get.vi"("refnum name"="Air Valve 2") -> ("error out"=w348:errorcluster, "SolenoidDevRef"=w345:T7)  [unwired: 9 in]
      n212 = call <vilib>:"WPI_SolenoidRefNum Registry Get.vi"("refnum name"="Air Valve 3") -> ("error out"=w331:errorcluster, "SolenoidDevRef"=w339:T7)  [unwired: 9 in]
      n213 = call <vilib>:"WPI_SolenoidRefNum Registry Get.vi"("refnum name"="Air Valve 6") -> ("error out"=w316:errorcluster, "SolenoidDevRef"=w319:T7)  [unwired: 9 in]
      n214 = call <vilib>:"WPI_SolenoidRefNum Registry Get.vi"("refnum name"="Air Valve 5") -> ("error out"=w323:errorcluster, "SolenoidDevRef"=w326:T7)  [unwired: 9 in]
      n215 = call <vilib>:"WPI_SolenoidRefNum Registry Get.vi"("refnum name"="Air Valve 4") -> ("error out"=w330:errorcluster, "SolenoidDevRef"=w334:T7)  [unwired: 9 in]
      n216 = call-poly <vilib>:"WPI_SolenoidSet.vi"("error in (no error)"=w355, "Value"=w350, "SolenoidDevRef"=w354) -> ()  [unwired: 7 in, 2 out]
      n217 = call-poly <vilib>:"WPI_SolenoidSet.vi"("error in (no error)"=w348, "Value"=w344, "SolenoidDevRef"=w345) -> ()  [unwired: 7 in, 2 out]
      n218 = call-poly <vilib>:"WPI_SolenoidSet.vi"("error in (no error)"=w331, "Value"=w337, "SolenoidDevRef"=w339) -> ()  [unwired: 7 in, 2 out]
      n219 = call-poly <vilib>:"WPI_SolenoidSet.vi"("error in (no error)"=w316, "Value"=w317, "SolenoidDevRef"=w319) -> ()  [unwired: 7 in, 2 out]
      n220 = call-poly <vilib>:"WPI_SolenoidSet.vi"("error in (no error)"=w323, "Value"=w324, "SolenoidDevRef"=w326) -> ()  [unwired: 7 in, 2 out]
      n221 = call-poly <vilib>:"WPI_SolenoidSet.vi"("error in (no error)"=w330, "Value"=w332, "SolenoidDevRef"=w334) -> ()  [unwired: 7 in, 2 out]
    }
    frame Disabled {
    }
  }
  n222 = disable-structure shown="Disabled" {
    frame Disabled {
      # "Intake"
      n223 = call <vilib>:"WPI_JoystickRefNum Registry Get.vi"("refnum name"="Right Stick") -> ("error out"=w375:errorcluster, "JoystickDevRef"=w374:T4)  [unwired: 9 in]
      n224 = call <vilib>:"WPI_JoystickGetValues.vi"("error in (no error)"=w375, "JoystickDevRef"=w374) -> ("Buttons"=w372:bool[])  [unwired: 5 in, 4 out]
      n225 = Array To Cluster(array=w372) -> (cluster=w371:T6)
      n226 = Unbundle By Name(w371) -> ("Buttons[4]"=w367:bool, "Buttons[2]"=w366:bool)
      n227 = Select(t=1.0, s=w367, f=0.0) -> (s? t:f=w363:dbl)
      n228 = Select(t=-1.0, s=w366, f=w363) -> (s? t:f=w361:dbl)
      n229 = call <vilib>:"WPI_MotorControlRefNum Registry Get.vi"("refnum name"="Intake") -> ("error out"=w369:errorcluster, "MotorControlDevRef"=w368:T12)  [unwired: 9 in]
      n230 = call <vilib>:"WPI_MotorControlSetOutput.vi"("error in (no error)"=w369, "Output"=w361, "MotorControlDevRef"=w368) -> ()  [unwired: 6 in, 3 out]
    }
    frame Enabled {
    }
  }
  n231 = call-poly <vilib>:"NT Read Value.vi"("Name"="DB/Button 0" ("refnum name")) -> ("Boolean"=→"Sample Boolean 0":bool)  [unwired: 9 in, 1 out]
  n232 = call-poly <vilib>:"NT Read Value.vi"("Name"="DB/Slider 0" ("refnum name")) -> ("Numeric"=→"Sample Slider 0":dbl)  [unwired: 9 in, 1 out]
  n233 = call-poly <vilib>:"NT Read Value.vi"("Name"="DB/Button 1" ("refnum name")) -> ("Boolean"=→"Sample Boolean 1":bool)  [unwired: 9 in, 1 out]
  n234 = call <vilib>:"WPI_CompressorRefNum Registry Get.vi"("refnum name"="Compressor") -> ("error out"=w1:errorcluster, "CompressorDevRef"=w2:T23)  [unwired: 9 in]
  n235 = call <vilib>:"WPI_CompressorGetEnableState.vi"("error in (no error)"=w1, "CompressorDevRef"=w2) -> ()  [unwired: 6 in, 4 out]
